vi "delete device group name.vi"(8 "error in (no error)":errorcluster, 11 "device group name":string) -> (0 "error out":errorcluster)   [LabVIEW 2018]
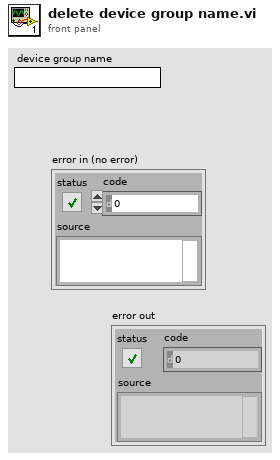
[diagram p1: front panel]
types:
  T1 = typedef "mysql_authentication.ctl" = cluster{"User":string, "Password":string, "Database":string}
  T2 = cluster{"Port":u16, "IP Address":string, "Authentication":T1}
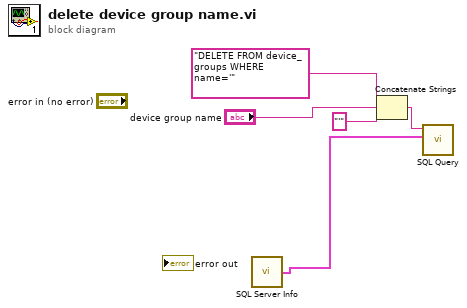
[diagram p0: block diagram]
diagram:
  n1 = call "SQL Server Info.vi"() -> ("SQL Server Info"=w2:T2)
  n2 = Concatenate Strings("DELETE FROM device_groups WHERE name='" ("message"), "device group name", "'" ("Query")) -> (w4:string)
  n3 = call "SQL Query.vi"("SQL Server Info"=w2, "Query"=w4) -> ()  [unwired: 8 in, 2 out]
